vi "Stop Core.vi"(10 "final error code":i32, 11 "MQTT-Client in":refnum<class "MQTT-Client.lvclass">) -> (3 "MQTT-Client out":refnum<class "MQTT-Client.lvclass">)   [LabVIEW 2023, in "MQTT-Client.lvlib" / "MQTT-Client.lvclass"]
doc: "(<B>Filename</B>: Actor Framework.lvlib:Actor.lvclass:Stop Core.vi)\n\nDefines what the actor does before it stops. Use the <B>final error code</B> input to determine whether the actor shut down in response to an error.\n\nBy default, this method passes the Stop message along to all auto-stop nested actors. A descendant class may override this method to define additional behavior, such as shutting down any processes the actor initiated in its override of the Actor Core method."
uses:
  MQTT-Client.lvclass
  MQTT-Client.lvclass/MQTT-Client.ctl
  <vilib>/ActorFramework/Actor/Actor.lvclass
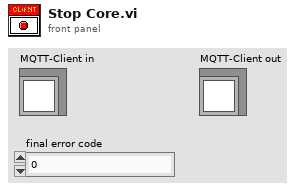
[diagram p1: front panel]
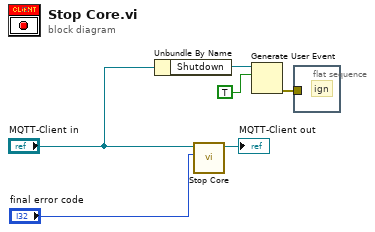
[diagram p0: block diagram]
diagram:
  n1 = Unbundle By Name("MQTT-Client in") -> ("Shutdown"=w4:refnum<user-event>)
  n2 = call-parent "Stop Core.vi"("final error code"="final error code", "Actor in"="MQTT-Client in") -> ("Actor out"=→"MQTT-Client out":refnum<class "MQTT-Client.lvclass">)  [unwired: 9 in]
  n3 = Generate User Event(user event=w4, event data cluster=TRUE ("event data")) -> (error out=w2:errorcluster)  [unwired: 2 in, 1 out]
  n4 = flat-sequence {
    tunnel: w2 -> [_]
    frame #0 {
      # "ign"
    }
  }
